vi "Circulo.vi"(10 "Paso":dbl, 11 "Tiempo":dbl) -> (2 "Y":dbl[](array[numeric]), 3 "X":dbl[](array[numeric]))   [LabVIEW 2011]
panel:
  out "XY Graph":cluster{dbl[], dbl[]}(graph)
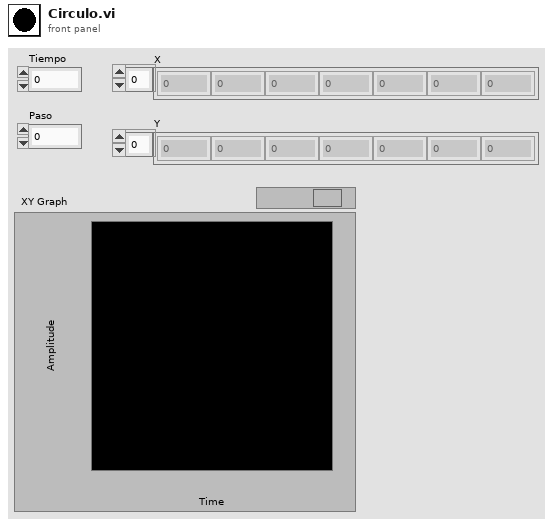
[diagram p1: front panel]
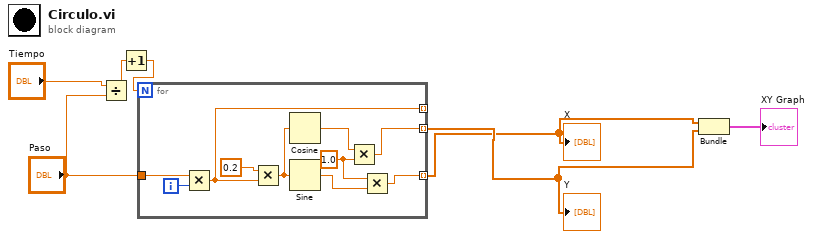
[diagram p0: block diagram]
diagram:
  n1 = Divide(x="Tiempo", y="Paso") -> (x/y=w4:dbl)
  n2 = Increment(x=w4) -> (x+1=w5:dbl)
  n3 = for {
    N: w5 -> [_]
    tunnel: [w11] -> w2 mode=indexing
    tunnel: [w8] -> w1 mode=indexing
    tunnel: "Paso" -> [w16]
    tunnel: [w13] -> _ mode=indexing
    i -> [w17]
    w10 = 1.0 ("y")
    n4 = Multiply(x=w16, y=w17) -> (x*y=w13:dbl)
    n5 = Multiply(x=0.2, y=w13) -> (x*y=w14:dbl)
    n6 = Cosine(x=w14) -> (cos(x)=w12:dbl)
    n7 = Sine(x=w14) -> (sin(x)=w9:dbl)
    n8 = Multiply(x=w12, y=w10) -> (x*y=w11:dbl)
    n9 = Multiply(x=w10, y=w9) -> (x*y=w8:dbl)
  }
  "Y" <- w2
  "X" <- w1
  n10 = Bundle(w1, w2) -> (→"XY Graph":cluster{dbl[], dbl[]})  [unwired: 1 in]
